vi "Take Snapshot.vi"(8 "error in":errorcluster, 11 "Instruments in":refnum<class "Instruments.lvclass">) -> (0 "error out":errorcluster, 3 "Instruments out":refnum<class "Instruments.lvclass">)   [LabVIEW 2023, in "Instruments.lvlib" / "Instruments.lvclass"]
uses:
  Library/Instruments.lvclass
  C:/Users/Public/Documents/Development/builds/Framework/Engine.lvlibp/Engine/Library/Engine.lvclass
  C:/Users/Public/Documents/Development/builds/Framework/Actor Framework.lvlibp/1abvi3w/vi.lib/ActorFramework/Actor/Actor.lvclass
  Library/Instruments.lvclass/Instruments.ctl
  builds/Framework/Engine.lvlibp/Engine/Accessors/Read Report Q.vi
  builds/Framework/Actor Framework.lvlibp/1abvi3w/vi.lib/ActorFramework/Actor/Read Actor Label.vi
  builds/Tools/QDMH.lvlibp/Private/Enqueue Single Element.vi
  builds/Tools/QDMH.lvlibp/Library/QDMH.lvclass
  builds/Framework/Engine.lvlibp/Engine/Library/Engine.lvclass
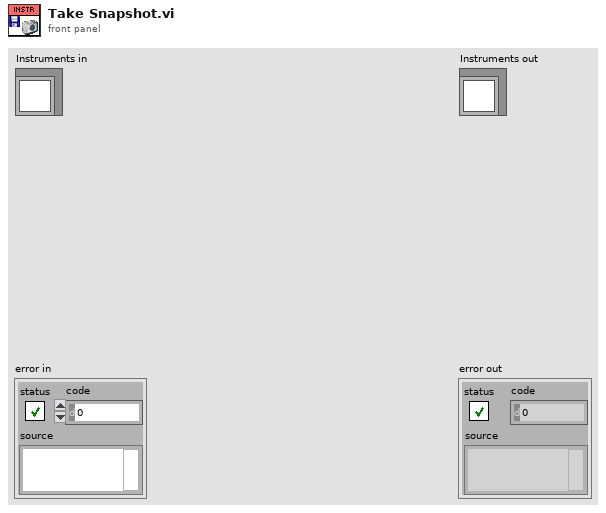
[diagram p1: front panel]
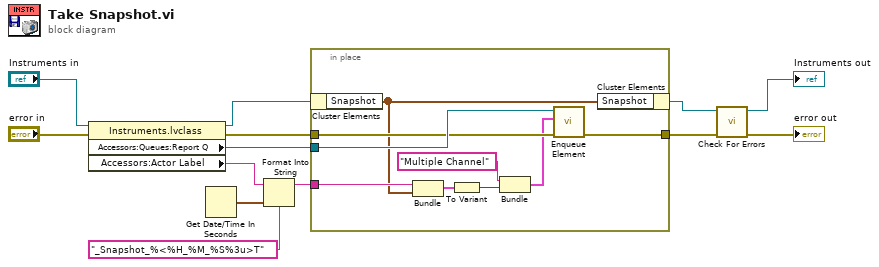
[diagram p0: block diagram]
diagram:
  n1 = property class="Instruments.lvclass"(reference="Instruments in", error in="error in") -> (reference out=w8:refnum<class "Instruments.lvclass">, error out=w6:errorcluster, "Accessors:Queues:Report Q"=w7:refnum<class "QDMH.lvclass">, "Accessors:Actor Label"=w9:string)
  n2 = Get Date/Time In Seconds() -> (seconds since 1Jan1904=w11:timestamp)
  n3 = Format Into String(format string="_Snapshot_%<%H_%M_%S%3u>T", initial string=w9, w11) -> (resulting string=w4:string)  [unwired: 1 in, 1 out]
  n4 = in-place {
    in-place-border: w7 -> [w22]
    in-place-border: w6 -> [w21]
    in-place-border: [w20] -> w5
    in-place-border: w4 -> [w15]
    n5 = in-place-cluster #1(w8) -> ("Snapshot"=w14:waveform(dbl)[])
    n6 = Bundle(w15, "Snapshot"=w14) -> (w17:cluster{string, "Snapshot":waveform(dbl)[]})  [unwired: 1 in]
    n7 = To Variant(anything=w17) -> (Variant=w16:variant)
    n8 = Bundle("Multiple Channel", "Variant"=w16) -> (w18:cluster{string, "Variant":variant})  [unwired: 1 in]
    n9 = call-poly "Enqueue Element.vi"("error in (no error)"=w21, "Message"=w18, "QDMH in"=w22) -> ("error out"=w20:errorcluster)  [unwired: 7 in, 1 out]
    n10 = in-place-cluster #1("Snapshot"=w14) -> (w2:refnum<class "Instruments.lvclass">)
  }
  n11 = call "Check For Errors.vi"("error in"=w5, "Engine in"=w2) -> ("error out"=→"error out":errorcluster, "Engine out"=→"Instruments out":refnum<class "Instruments.lvclass">)  [unwired: 8 in]
